vi "PythonWrapper.vi"(0 "file to run":path, 1 "expected output size (4096)":u32=4096, 2 "Python.exe":path=path "Python", 3 "data in":variant, 4 "run minimized? (T)":bool=TRUE) -> (5 "data out":variant, 6 "standard error":string, 7 "return code":i32, 8 "error out":errorcluster)   [LabVIEW 2016]
doc: "Allows for the passing of non-string data types to and from Python scripts."
uses:
  <vilib>/Utility/error.llb/DialogType.ctl
panel:
  in  "Show More":bool
  out "Flattened Output":string
  out "Flattened Input":string
  out "Raw Input":string
  out "Raw Output":string
  # "INPUTS"
  # "OUTPUTS"
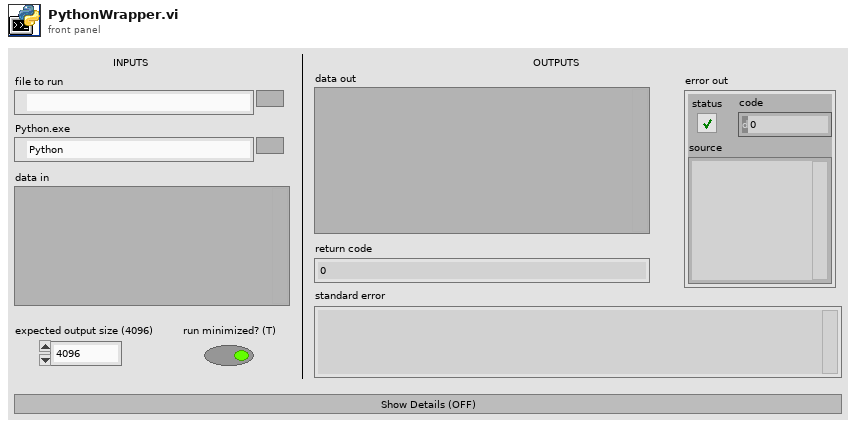
[diagram p1: front panel]
types:
  T1 = enum16{"big-endian, network order", "native, host order", "little-endian"}
  T2 = typedef "DialogType.ctl" = u16
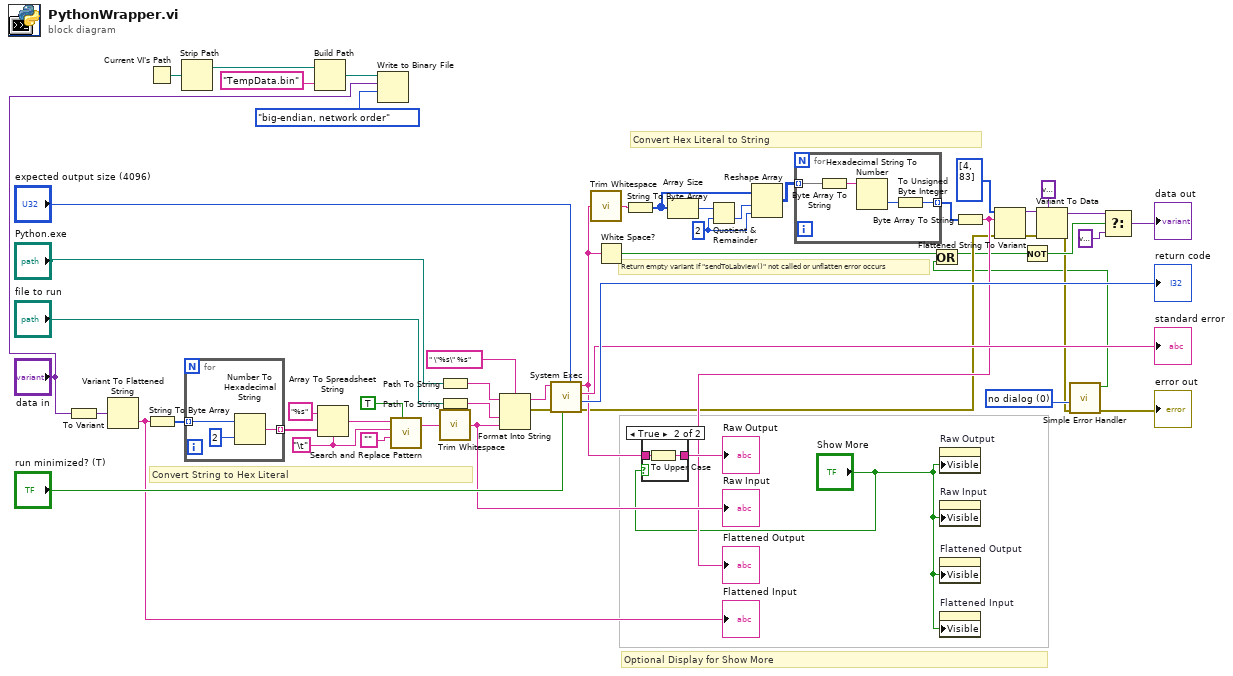
[diagram p0: block diagram]
diagram:
  w13 = T2 0 items=["no dialog", "OK message", "continue or stop message", "OK message + warnings", "continue/stop + warnings"] ("type of dialog (OK msg:1)")
  w33 = 2
  w50 = "\t"
  # "Return empty variant if \"sendToLabview()\" not called or unflatten error occurs"
  # "Convert Hex Literal to String"
  # "Optional Display for Show More"
  # "Convert String to Hex Literal"
  n1 = To Variant(anything="data in") -> (Variant=w54:variant)
  n2 = Variant To Flattened String(Variant=w54) -> (data string=w24:string)  [unwired: 1 out]
  "Flattened Input" <- w24
  n3 = Current VI's Path() -> (path=w5:path)
  n4 = String To Byte Array(string=w24) -> (unsigned byte array=w53:u8[])
  n5 = Strip Path(path=w5) -> (stripped path=w4:path)  [unwired: 1 out]
  n6 = for {
    tunnel: w53 -> [w56] mode=indexing
    tunnel: [w55] -> w46 mode=indexing
    n7 = Number To Hexadecimal String(1:2, 2:w56) -> (0:w55:string)
  }
  n8 = Build Path(base path=w4, name or relative path="TempData.bin") -> (appended path=w3:path)
  n9 = Array To Spreadsheet String(delimiter (Tab)=w50, array=w46, 3:"%s") -> (spreadsheet string=w51:string)
  n10 = Write to Binary File(file (use dialog)=w3, data="data in", 9:T1."big-endian, network order" ("byte order (0:big-endian, network order)")) -> ()  [unwired: 3 in, 3 out]
  n11 = call <vilib>:"Search and Replace Pattern.vi"("string"=w51, "regular expression (\"\")"=w50, "replace string (\"\")"="", "replace all? (F)"=TRUE) -> ("result string"=w47:string)  [unwired: 1 in, 1 out]
  n12 = Path To String(path="Python.exe") -> (string=w45:string)
  n13 = Path To String(path="file to run") -> (string=w44:string)
  n14 = call <vilib>:"Trim Whitespace.vi"("string"=w47) -> ("trimmed string"=w25:string)  [unwired: 1 in]
  "Raw Input" <- w25
  n15 = Format Into String(format string=" \"%s\" %s", initial string=w45, w44, w25) -> (resulting string=w41:string, error out=w42:errorcluster)  [unwired: 1 in]
  n16 = call <vilib>:"System Exec.vi"("expected output size  (4096)"="expected output size (4096)", "run minimized? (F)"="run minimized? (T)", "error in (no error)"=w42, "command line"=w41) -> ("error out"=w10:errorcluster, "return code"=→"return code":i32, "standard error"=→"standard error":string, "standard output"=w14:string)  [unwired: 4 in]
  n17 = call <vilib>:"Trim Whitespace.vi"("string"=w14) -> ("trimmed string"=w20:string)  [unwired: 1 in]
  n18 = White Space?(1:w14) -> (0:w15:bool)
  n19 = String To Byte Array(string=w20) -> (unsigned byte array=w31:u8[])
  n20 = case shown="True" "Show More" {
    tunnel: w14 -> [w58 w60]
    tunnel: [w58 w59] -> w23
    frame False {
    }
    frame True {
      n21 = To Upper Case(1:w60) -> (0:w59:string)
    }
  }
  "Raw Output" <- w23
  n22 = Array Size(array=w31) -> (size(s)=w32:i32)
  n23 = Quotient & Remainder(x=w32, y=w33) -> (floor(x/y)=w34:i32)  [unwired: 1 out]
  n24 = Reshape Array(w31, w34, w33) -> (w30:u8[][])
  n25 = for {
    tunnel: w30 -> [w61] mode=indexing
    tunnel: [w62] -> w29 mode=indexing
    n26 = Byte Array To String(unsigned byte array=w61) -> (string=w64:string)
    n27 = Hexadecimal String To Number(string=w64) -> (number=w63:u32)  [unwired: 2 in, 1 out]
    n28 = To Unsigned Byte Integer(number=w63) -> (unsigned 8bit integer=w62:u8)
  }
  n29 = property on="Raw Output" class="Str"("Visible"="Show More") -> ()  [unwired: 2 in, 2 out]
  n30 = property on="Raw Input" class="Str"("Visible"="Show More") -> ()  [unwired: 2 in, 2 out]
  n31 = property on="Flattened Output" class="Str"("Visible"="Show More") -> ()  [unwired: 2 in, 2 out]
  n32 = property on="Flattened Input" class="Str"("Visible"="Show More") -> ()  [unwired: 2 in, 2 out]
  n33 = Byte Array To String(unsigned byte array=w29) -> (string=w22:string)
  "Flattened Output" <- w22
  n34 = Flattened String To Variant(4:w10, 6:w22, 7:i16[] [4, 83]) -> (0:w11:errorcluster, 3:w36:variant)
  n35 = Variant To Data(error in=w11, type=variant, Variant=w36) -> (data=w18:variant, error out=w12:errorcluster)
  n36 = call <vilib>:"Simple Error Handler.vi"("type of dialog (OK msg:1)"=w13, "error in (no error)"=w12) -> ("error?"=w7:bool, "error out"=→"error out":errorcluster)  [unwired: 3 in, 3 out]
  n37 = Or(x=w15, y=w7) -> (x .or. y?=w8:bool)
  n38 = Not(x=w8) -> (.not. x?=w16:bool)
  n39 = Select(t=w18, s=w16, f=variant) -> (s? t:f=→"data out":variant)
